vi "ReplaceErrorConnectID.vi"(8 "ConnectArrayIN":T1(array[cluster]), 10 "ErrorIN":errorcluster, 11 "ConnectID":refnum<k5>) -> (0 "ConnectArrayOUT":T1(array[cluster]))   [LabVIEW 2011]
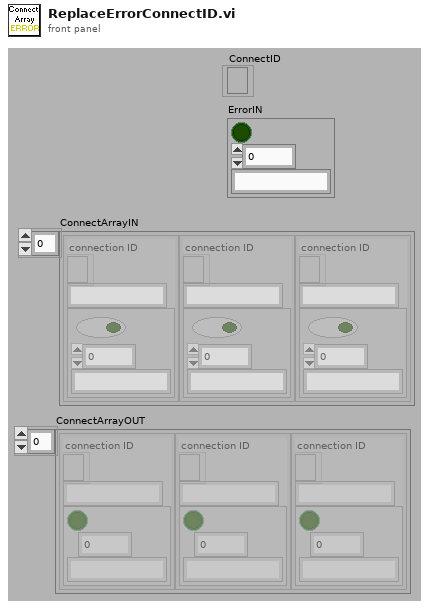
[diagram p1: front panel]
types:
  T1 = cluster{"connection ID":refnum<k5>, string, errorcluster}[]
  T2 = cluster{"ConnectID":refnum<k5>, string, "ErrorIN":errorcluster}
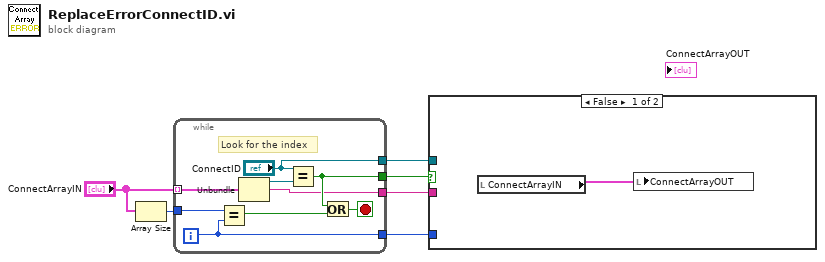
[diagram p0: block diagram]
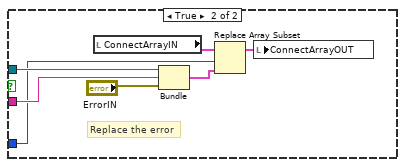
[diagram p2: hidden frame]
diagram:
  n1 = Array Size(array="ConnectArrayIN") -> (size(s)=w5:i32)
  n2 = while {
    tunnel: "ConnectArrayIN" -> [w15] mode=indexing
    tunnel: w5 -> [w12]
    tunnel: [w10] -> w4
    tunnel: [w9] -> w3
    tunnel: [w8] -> w2
    tunnel: ["ConnectID"] -> w1
    i -> [w9]
    stop <- w11 stop-if-true
    # "Look for the index"
    n3 = Equal?(x=w12, y=w9) -> (x = y?=w13:bool)
    n4 = Unbundle(w15) -> ("connection ID"=w14:refnum<k5>, w8:string)  [unwired: 1 out]
    n5 = Equal?(x="ConnectID", y=w14) -> (x = y?=w10:bool)
    n6 = Or(x=w10, y=w13) -> (x .or. y?=w11:bool)
  }
  n7 = case shown="False" w4 {
    tunnel: w3 -> [_ w19]
    tunnel: w2 -> [_ w22]
    tunnel: w1 -> [_ w21]
    frame False {
      n8 = local read "ConnectArrayIN"() -> (w16:T1)
      n9 = local write "ConnectArrayOUT"(w16) -> ()
    }
    frame True {
      # "Replace the error"
      n10 = local read "ConnectArrayIN"() -> (w23:T1)
      n11 = Bundle("ConnectID"=w21, w22, "ErrorIN"="ErrorIN") -> (w20:T2)  [unwired: 1 out]
      n12 = Replace Array Subset(array=w23, new element=w20, index=w19) -> (w17:T1)
      n13 = local write "ConnectArrayOUT"(w17) -> ()
    }
  }
